vi "Limelight Base Speed Calculator.vi"(11 "Limelight TA":dbl) -> (3 "Base Drive Speed":dbl)   [LabVIEW 2018]
uses:
  Robot Global Data.vi
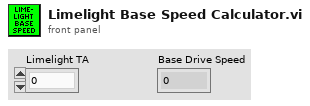
[diagram p1: front panel]
types:
  T1 = typedef "Which Robot Enum.ctl" = enum16{"Competition Bot", "Practice Bot", "Code Bot"}
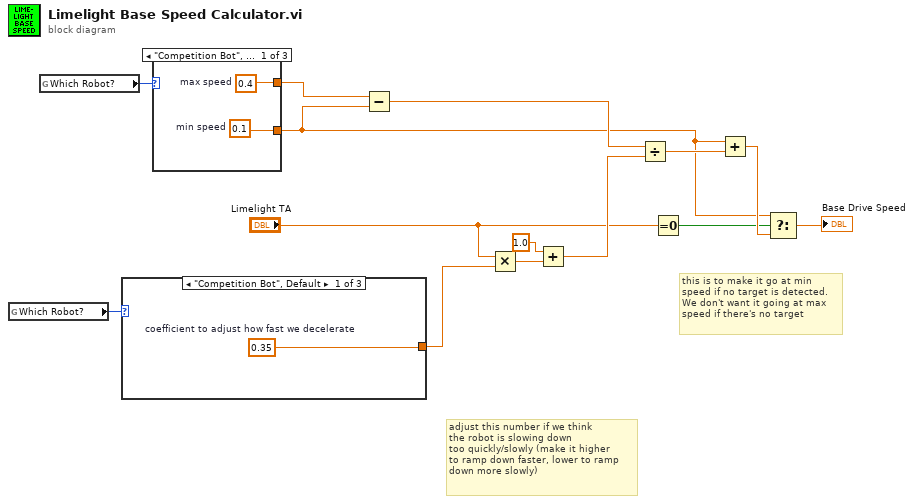
[diagram p0: block diagram]
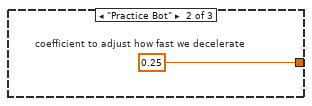
[diagram p2: hidden frame]
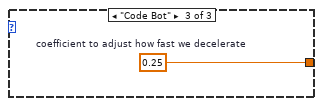
[diagram p3: hidden frame]
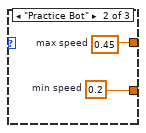
[diagram p4: hidden frame]
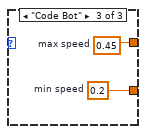
[diagram p5: hidden frame]
diagram:
  # "this is to make it go at min\nspeed if no target is detected.\nWe don't want it going at max\nspeed if there's no target"
  # "adjust this number if we think\nthe robot is slowing down\ntoo quickly/slowly (make it higher\nto ramp down faster, lower to ramp\ndown more slowly)"
  n1 = global read "Robot Global Data.vi" "Which Robot?"() -> (w2:T1)
  n2 = global read "Robot Global Data.vi" "Which Robot?"() -> (w9:T1)
  n3 = case shown="\"Competition Bot\", Default" w2 {
    tunnel: [w15 w16 w17] -> w1
    frame "Competition Bot", Default {
      w15 = 0.35  # coefficient to adjust how fast we decelerate
    }
    frame "Practice Bot" {
      w16 = 0.25  # coefficient to adjust how fast we decelerate
    }
    frame "Code Bot" {
      w17 = 0.25  # coefficient to adjust how fast we decelerate
    }
  }
  n4 = case shown="\"Competition Bot\", Default" w9 {
    tunnel: [w19 w21 w23] -> w8
    tunnel: [w18 w20 w22] -> w3
    frame "Competition Bot", Default {
      w19 = 0.4  # max speed
      w18 = 0.1  # min speed
    }
    frame "Practice Bot" {
      w21 = 0.45  # max speed
      w20 = 0.2  # min speed
    }
    frame "Code Bot" {
      w23 = 0.45  # max speed
      w22 = 0.2  # min speed
    }
  }
  n5 = Subtract(x=w8, y=w3) -> (x-y=w12:dbl)
  n6 = Multiply(x="Limelight TA", y=w1) -> (x*y=w14:dbl)
  n7 = Add(x=1.0, y=w14) -> (x+y=w11:dbl)
  n8 = Divide(x=w12, y=w11) -> (x/y=w10:dbl)
  n9 = Equal To 0?(x="Limelight TA") -> (x = 0?=w5:bool)
  n10 = Add(x=w3, y=w10) -> (x+y=w6:dbl)
  n11 = Select(t=w3, s=w5, f=w6) -> (s? t:f=→"Base Drive Speed":dbl)
